vi "readInCSVFile.vi"(8 "error in":errorcluster, 10 "Path":path=path "C:/Users/Administrator/Desktop/Crete/Data/2014/1411/141126/Scripts/Instrument Scripts/Dio64.csv") -> (0 "error out":errorcluster, 1 "Array":dbl[][](array[numeric]), 2 "channels":string)   [LabVIEW 2011, in "run.lvlib"]
uses:
  run.lvlib
panel:
  out "device":string
  out "Configuration":string[](array[string])
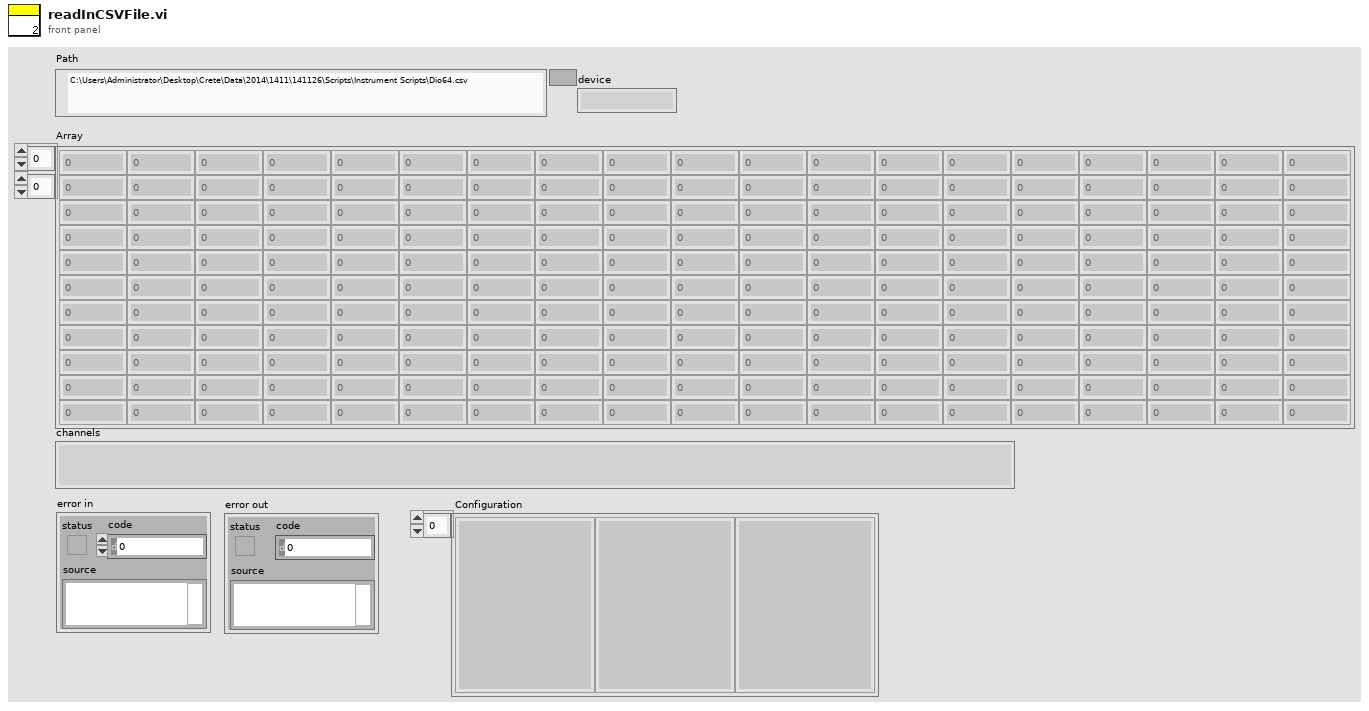
[diagram p1: front panel]
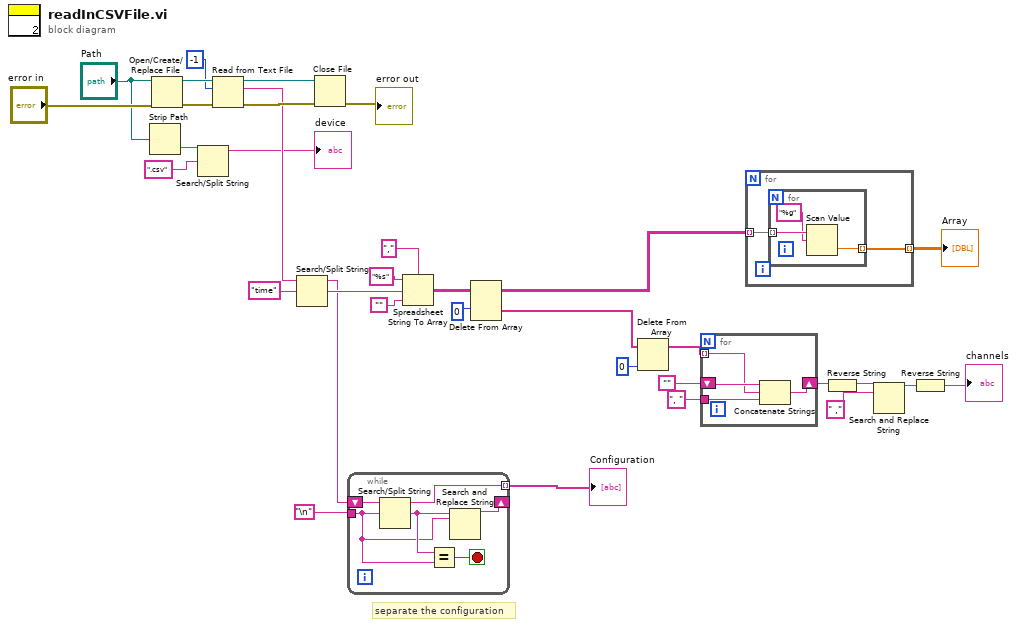
[diagram p0: block diagram]
diagram:
  # "separate the configuration"
  n1 = Strip Path(path="Path") -> (name=w3:string)  [unwired: 1 out]
  n2 = Open/Create/Replace File(file path (use dialog)="Path", error in="error in") -> (refnum out=w32:refnum<file>, error out=w14:errorcluster)  [unwired: 4 in, 1 out]
  n3 = Search/Split String(string=w3, search string/char (-)=".csv") -> (substring before match=→"device":string)  [unwired: 1 in, 2 out]
  n4 = Read from Text File(file (use dialog)=w32, count=-1, error in=w14) -> (refnum out=w31:refnum<file>, text=w10:string, error out=w15:errorcluster)  [unwired: 1 in, 1 out]
  n5 = Search/Split String(string=w10, search string/char (-)="time") -> (substring before match=w7:string, match + rest of string=w9:string)  [unwired: 1 in, 1 out]
  n6 = Close File(refnum=w31, error in=w15) -> (error out=→"error out":errorcluster)  [unwired: 1 out]
  n7 = while {
    tunnel: "\n" -> [w35]
    shift-right: [w36] -> _
    shift-left: w7 -> [w40]
    tunnel: [w39] -> w5 mode=indexing
    stop <- w38 stop-if-true
    n8 = Search/Split String(string=w40, search string/char (-)=w35) -> (substring before match=w39:string, match + rest of string=w37:string)  [unwired: 1 in, 1 out]
    n9 = Equal?(x=w37, y=w35) -> (x = y?=w38:bool)
    n10 = Search and Replace String(input string=w37, search string=w35) -> (result string=w36:string)  [unwired: 6 in, 3 out]
  }
  "Configuration" <- w5
  n11 = Spreadsheet String To Array(delimiter (Tab)=",", format string="%s", spreadsheet string=w9, array type (2D Dbl)="") -> (array=w11:string[][])
  n12 = Delete From Array(array=w11, index (row)=0) -> (deleted portion=w21:string[], array with subset deleted=w18:string[][])  [unwired: 2 in]
  n13 = Delete From Array(array=w21, index=0) -> (array with subset deleted=w20:string[])  [unwired: 1 in, 1 out]
  n14 = for {
    tunnel: w20 -> [w43] mode=indexing
    shift-right: [w42] -> w26
    shift-left: "" -> [w44]
    tunnel: ", " -> [w41]
    n15 = Concatenate Strings(w44, w43, w41) -> (w42:string)
  }
  n16 = for {
    tunnel: w18 -> [w46] mode=indexing
    tunnel: [w45] -> w17 mode=indexing
    n17 = for {
      tunnel: w46 -> [w49] mode=indexing
      tunnel: [w47] -> w45 mode=indexing
      n18 = Scan Value(string=w49, format string="%g") -> (value=w47:dbl)  [unwired: 1 in, 1 out]
    }
  }
  "Array" <- w17
  n19 = Reverse String(1:w26) -> (0:w25:string)
  n20 = Search and Replace String(input string=w25, search string=" ,") -> (result string=w23:string)  [unwired: 6 in, 3 out]
  n21 = Reverse String(1:w23) -> (0:→"channels":string)
